vi "Czy _wybrano_stala.vi"(7 "output cluster":T2, 9 "Przebieg C":i32, 10 "Przebieg B":i32, 11 "Przebieg A":i32) -> (0 "akcja":u8, 1 "Stala C?":bool, 2 "Stala B?":bool, 3 "Stala A?":bool)   [LabVIEW 2013]
doc: "Sprawdza czy na kanalach A B C\nwybrano przebieg czy stałą"
uses:
  <vilib>/Utility/miscctls.llb/LVStringsAndValuesArrayTypeDef_I32.ctl
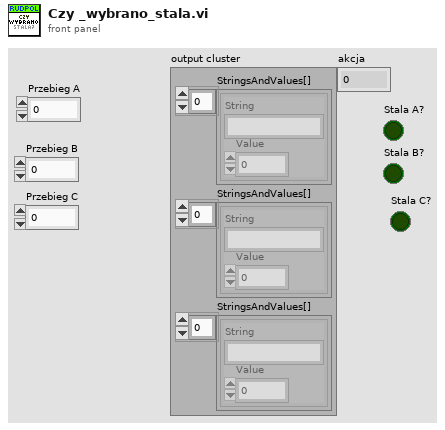
[diagram p1: front panel]
types:
  T1 = typedef "LVStringsAndValuesArrayTypeDef_I32.ctl" = cluster{"String":string, "Value":i32}[]
  T2 = cluster{"StringsAndValues[]":T1, "StringsAndValues[]":T1, "StringsAndValues[]":T1}
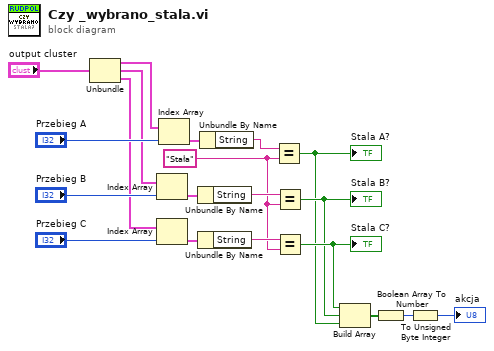
[diagram p0: block diagram]
diagram:
  w9 = "Stała"
  n1 = Unbundle("output cluster") -> ("StringsAndValues[]"=w11:T1, "StringsAndValues[]"=w8:T1, "StringsAndValues[]"=w7:T1)
  n2 = Index Array(array=w8, index="Przebieg B") -> (element=w15:cluster{"String":string, "Value":i32})
  n3 = Index Array(array=w7, index="Przebieg C") -> (element=w13:cluster{"String":string, "Value":i32})
  n4 = Index Array(array=w11, index="Przebieg A") -> (element=w18:cluster{"String":string, "Value":i32})
  n5 = Unbundle By Name(w15) -> ("String"=w16:string)
  n6 = Unbundle By Name(w13) -> ("String"=w12:string)
  n7 = Unbundle By Name(w18) -> ("String"=w17:string)
  n8 = Equal?(x=w17, y=w9) -> (x = y?=w4:bool)
  "Stala A?" <- w4
  n9 = Equal?(x=w16, y=w9) -> (x = y?=w5:bool)
  "Stala B?" <- w5
  n10 = Equal?(x=w12, y=w9) -> (x = y?=w6:bool)
  "Stala C?" <- w6
  n11 = Build Array(w6, w5, w4) -> (w3:bool[])
  n12 = Boolean Array To Number(Boolean array=w3) -> (number=w2:u32)
  n13 = To Unsigned Byte Integer(number=w2) -> (unsigned 8bit integer=→"akcja":u8)
